vi "Event Structure Support in LabVIEW Real-Time.vi"(11 "reference":refnum<vi>) -> ()   [LabVIEW 2019]
panel:
  out "Numeric Indicator within Event 2":i32
  in  "stop 2":bool
  out "event loop iteration 2":i32
  out "Event Registration Refnum":refnum<event-registration>
  out "Boolean":bool
  out "Numeric Indicator within Event":i32
  in  "stop":bool
  out "event loop iteration":i32
  out "error out":errorcluster
  in  "Numeric":i32
  out "nonevent loop iteration":i32
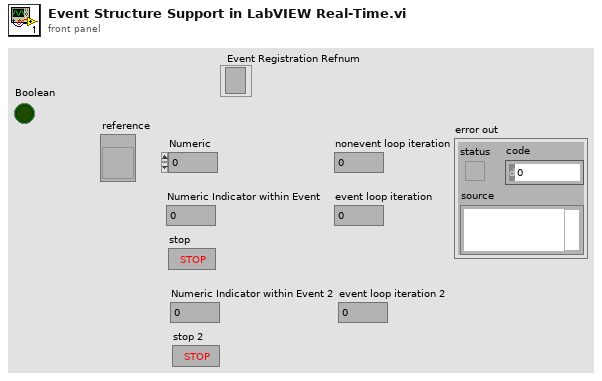
[diagram p1: front panel]
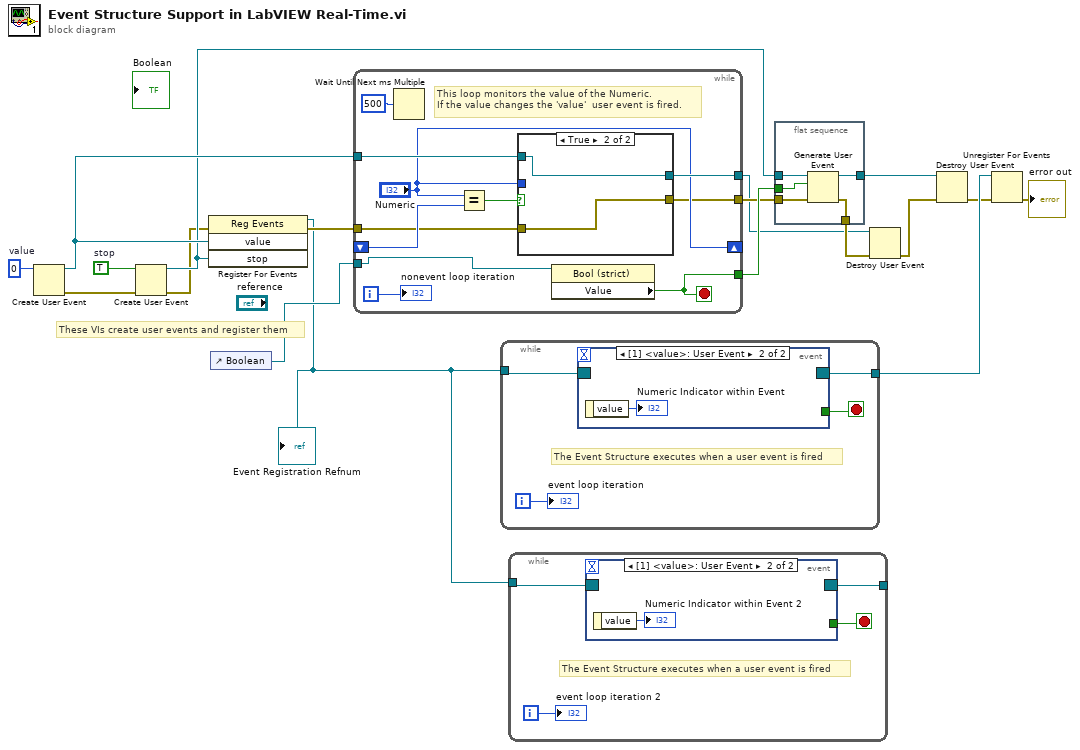
[diagram p0: block diagram]
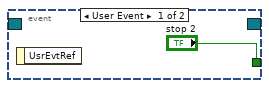
[diagram p2: hidden frame]
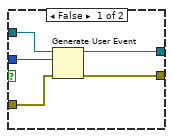
[diagram p3: hidden frame]
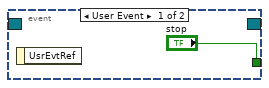
[diagram p4: hidden frame]
diagram:
  w14 = TRUE  # stop
  w17 = 0  # value
  # "These VIs create user events and register them"
  n1 = Create User Event(user event datatype=w17) -> (user event=w18:refnum<user-event>, error out=w8:errorcluster)  [unwired: 1 in]
  n2 = Create User Event(user event datatype=w14, error in=w8) -> (user event=w13:refnum<user-event>, error out=w7:errorcluster)
  n3 = register-events(error in=w7, w18, w13) -> (reference out=w1:refnum<event-registration>, error out=w6:errorcluster)  [unwired: 1 in]
  "Event Registration Refnum" <- w1
  n4 = control-ref of="Boolean"() -> (w2:refnum<vi>)
  n5 = while {
    shift-right: ["Numeric"] -> _
    shift-left: _ -> [w26]
    tunnel: w18 -> [w25]
    tunnel: [w24] -> w3
    tunnel: [w23] -> w9
    tunnel: w6 -> [w21]
    tunnel: [w20] -> w5
    tunnel: w2 -> [w19]
    i -> [w27]
    stop <- w23 stop-if-true
    # "This loop monitors the value of the Numeric.\nIf the value changes the 'value'  user event is fired."
    n6 = Wait Until Next ms Multiple(millisecond multiple=u32 500) -> ()  [unwired: 1 out]
    n7 = Equal?(x="Numeric", y=w26) -> (x = y?=w28:bool)
    n8 = case shown="True" w28 {
      tunnel: "Numeric" -> [w33 _]
      tunnel: w25 -> [w34 w36]
      tunnel: [w32 w36] -> w24
      tunnel: w21 -> [w31 w35]
      tunnel: [w30 w35] -> w20
      frame False {
        n9 = Generate User Event(user event=w34, event data cluster=w33, error in=w31) -> (user event out=w32:refnum<user-event>, error out=w30:errorcluster)  [unwired: 1 in]
      }
      frame True {
      }
    }
    n10 = property class="Bool (strict)"(reference=w19) -> ("Value"=w23:bool)  [unwired: 1 in, 2 out]
    "nonevent loop iteration" <- w27
  }
  n11 = while {
    tunnel: w1 -> [w38]
    tunnel: [w37] -> w16
    i -> [w39]
    stop <- w40 stop-if-true
    # "The Event Structure executes when a user event is fired"
    n12 = event shown="[1] <value>: User Event" {
      selector: w38 -> [_ _]
      dyn-events: [_ _] -> w37
      timeout: _ -> [_ _]
      tunnel: ["stop" _] -> w40
      event User Event {
        n13 = event-data() -> ()  [unwired: 1 in, 1 out]
      }
      event User Event {
        n14 = event-data() -> ("value"=→"Numeric Indicator within Event":i32)  [unwired: 1 in]
      }
    }
    "event loop iteration" <- w39
  }
  n15 = while {
    tunnel: w1 -> [w44]
    tunnel: [w43] -> _
    i -> [w45]
    stop <- w46 stop-if-true
    # "The Event Structure executes when a user event is fired"
    n16 = event shown="[1] <value>: User Event" {
      selector: w44 -> [_ _]
      dyn-events: [_ _] -> w43
      timeout: _ -> [_ _]
      tunnel: ["stop 2" _] -> w46
      event User Event {
        n17 = event-data() -> ()  [unwired: 1 in, 1 out]
      }
      event User Event {
        n18 = event-data() -> ("value"=→"Numeric Indicator within Event 2":i32)  [unwired: 1 in]
      }
    }
    "event loop iteration 2" <- w45
  }
  n19 = flat-sequence {
    tunnel: w13 -> [w53]
    tunnel: [w52] -> w10
    tunnel: w9 -> [w51]
    tunnel: w5 -> [w50]
    tunnel: [w49] -> w4
    frame #0 {
      n20 = Generate User Event(user event=w53, event data cluster=w51, error in=w50) -> (user event out=w52:refnum<user-event>, error out=w49:errorcluster)  [unwired: 1 in]
    }
  }
  n21 = Destroy User Event(user event=w3, error in=w4) -> (error out=w12:errorcluster)
  n22 = Destroy User Event(user event=w10, error in=w12) -> (error out=w11:errorcluster)
  n23 = Unregister For Events(event registration refnum=w16, error in=w11) -> (error out=→"error out":errorcluster)
